vi "sta_initialize(SubVI).vi"(11 "python version":T2=enum."3.6") -> (3 "클러스터":T1)   [LabVIEW 2018]
uses:
  Program Files (x86)/National Instruments/LabVIEW 2018/examples/Connectivity/Python/support/PythonVersionsEnum.ctl
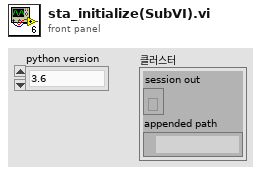
[diagram p1: front panel]
types:
  T1 = cluster{"session out":refnum<k35>, "appended path":path}
  T2 = typedef "PythonVersionsEnum.ctl" = enum16{"2.7", "3.6"}
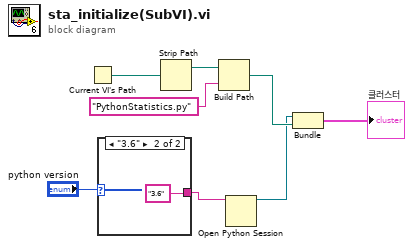
[diagram p0: block diagram]
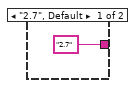
[diagram p2: hidden frame]
diagram:
  n1 = Current VI's Path() -> (path=w4:path)
  n2 = case shown="\"3.6\"" "python version" {
    tunnel: ["2.7" ("python version") "3.6" ("python version")] -> w8
    frame "2.7", Default {
    }
    frame "3.6" {
    }
  }
  n3 = Strip Path(path=w4) -> (stripped path=w3:path)  [unwired: 1 out]
  n4 = Build Path(base path=w3, name or relative path="PythonStatistics.py") -> (appended path=w2:path)
  n5 = Open Python Session(python version=w8) -> (session out=w1:refnum<k35>)  [unwired: 2 in, 1 out]
  n6 = Bundle("session out"=w1, "appended path"=w2) -> (→"클러스터":T1)  [unwired: 1 in]
